vi "New Results.vi"(7 "Image Nr.":i32, 8 "error in (no error)":errorcluster, 9 "Results In":refnum<class "Analyze Results Base.lvclass">[](array[class]), 10 "Parameters":refnum<class "Analyze Parameter Base.lvclass">[](array[class]), 11 "HIJ Single Cam App Demo In":refnum<class "HIJ Vision Camera App w Timer.lvclass">) -> (0 "error out":errorcluster, 3 "HIJ Single Cam App Demo Out":refnum<class "HIJ Vision Camera App w Timer.lvclass">)   [LabVIEW 2014, in "HIJ Vision Camera App w Timer.lvlib" / "HIJ Vision Camera App w Timer.lvclass"]
uses:
  HIJ Vision Camera App w Timer.lvclass
  Analyze/Results and Overlays/Results Base/Analyze Results Base.lvclass
  Analyze/Analyze Parameter/Analyze Parameter Base/Analyze Parameter Base.lvclass
  <vilib>/ActorFramework/Time-Delayed Send Message/Time-Delay Override Options.ctl
  HIJ Vision Camera App w Timer.lvclass/HIJ Vision Camera App w Timer.ctl
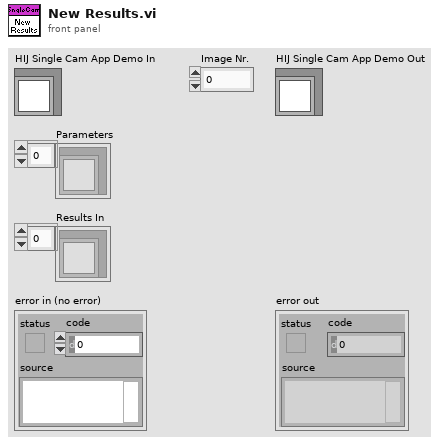
[diagram p1: front panel]
types:
  T1 = typedef "Time-Delay Override Options.ctl" = enum16{"Send next copy now", "Skip next scheduled copy", "Send next copy now and stop all further copies", "Stop all further copies"}
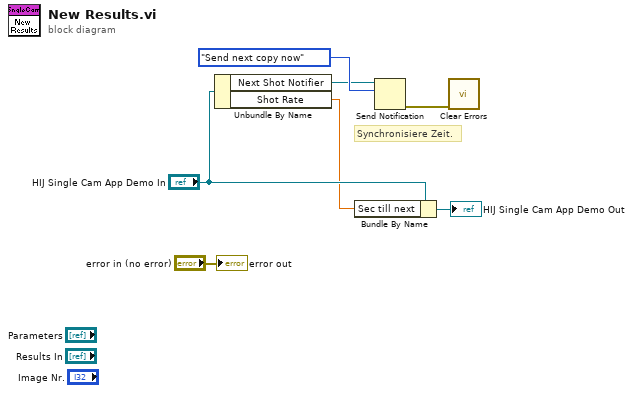
[diagram p0: block diagram]
diagram:
  # "Synchronisiere Zeit."
  n1 = Unbundle By Name("HIJ Single Cam App Demo In") -> ("Next Shot Notifier"=w3:refnum<notifier>, "Shot Rate"=w2:dbl)
  n2 = Bundle By Name(cluster="HIJ Single Cam App Demo In", "Sec till next"=w2) -> (→"HIJ Single Cam App Demo Out":refnum<class "HIJ Vision Camera App w Timer.lvclass">)
  n3 = Send Notification(notification=Time-Delay_Override_Options."Send next copy now", notifier=w3) -> (error out=w5:errorcluster)  [unwired: 1 in, 1 out]
  n4 = call <vilib>:"Clear Errors.vi"("error in (no error)"=w5) -> ()  [unwired: 5 in, 2 out]
  "error out" <- "error in (no error)"
